vi "Status Message.vi"(11 "?":string) -> ()   [LabVIEW 2021]
panel:
  out "?":string
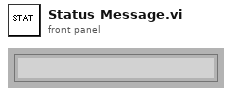
[diagram p1: front panel]
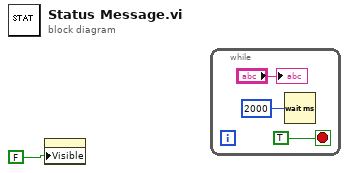
[diagram p0: block diagram]
diagram:
  n1 = property class="Str"("Visible"=FALSE) -> ()  [unwired: 2 in, 2 out]
  n2 = while {
    stop <- TRUE stop-if-true
    n3 = Wait (ms)(milliseconds to wait=u32 2000) -> ()  [unwired: 1 out]
    "?" <- "?"
  }
